vi "Arbitrary Shape Lowpass Filter Design.vi"() -> ()   [LabVIEW 2023]
doc: "Demonstrates how to design an arbitraty shape lowpass filter with two different methods. This example uses the DFD Remez Design VI to design a finite impulse response (FIR) arbitrary shape filter. This example also uses the DFD Least Pth Norm Design VI to design an infinite impulse response (IIR) arbitraty shape filter. You can see that the two filter designs are approximating the same ideal magnitude response.\n\nComplete the following steps to use this VI.\n1) Verify that this VI shows the <B>Remez Method</B> page.\n2) Run the VI and observe the magnitude response.\n3) Switch to the <B>Least Pth Norm Method</B> page.\n4) Run the VI again and observe the new magnitude response. Notice that the new magnitude response is similar to the previous one.\n5) Compare the specification settings on the <B>Remez Method</B> and <B>Least Pth Norm Method</B> pages and learn how to specify the same ideal magnitude response for different filter design methods."
uses:
  <vilib>/addons/Digital Filter Design/_LpNorm.llb/dfd_Lp Norm Filter Type.ctl
  <vilib>/addons/Digital Filter Design/_Objects.llb/DFD Adv Band Spec.ctl
  <vilib>/addons/Digital Filter Design/_REMEZ.llb/remez_fir filter type.ctl
  <vilib>/addons/Digital Filter Design/Design.llb/DFD Least Pth Norm Design by Newton.vi
  <vilib>/addons/Digital Filter Design/Analysis.llb/DFD Plot Freq Response (Linear-Spaced).vi
  <vilib>/addons/Digital Filter Design/NI_DigFilterLicensed.lvlib
panel:
  out "Error Message":string
  in  "Tab Control":enum32{"Remez Method", "Least Pth Norm Method"}(tab)
  in  "Sampling Frequency [Hz]":dbl=1.0 format="%.2f"
  in  "Filter Type":T1=enum."Minimum Phase"
  in  "Order":i32=40
  in  "Band Specifications":T2[](array[typedef])=[{"band specification"=[{"freq"=0.0, "amplitude"=1.0, "weight"=1.0}, {"freq"=0.1, "amplitude"=2.0, "weight"=1.0}, {"freq"=0.25, "amplitude"=1.0, "weight"=1.0}], "ripple constraint"=0.0}, {"band specification"=[{"freq"=0.3, "amplitude"=0.0, "weight"=1.0}, {"freq"=0.5, "amplitude"=0.0, "weight"=1.0}], "ripple constraint"=0.0}]
  in  "Band Specifications":T3(array[cluster])=[{"frequency point"=[{"frequency"=0.0, "magnitude"=1.0, "weight"=1.0, "phase"=0.0}, {"frequency"=0.1, "magnitude"=2.0, "weight"=1.0, "phase"=0.0}, {"frequency"=0.25, "magnitude"=1.0, "weight"=1.0, "phase"=0.0}]}, {"frequency point"=[{"frequency"=0.3, "magnitude"=0.0, "weight"=1.0, "phase"=0.0}, {"frequency"=0.5, "magnitude"=0.0, "weight"=1.0, "phase"=0.0}]}] {"frequency point"."weight" format="%.2f"}
  in  "Order":cluster{"numerator":i32, "denominator":i32}={"numerator"=8, "denominator"=8}
  in  "Filter Type":T4=enum."Minimum Phase"
  in  "Sampling Frequency [Hz]":dbl=1.0 format="%.2f"
  out "Magnitude Response":cluster{"f0":dbl, "df":dbl, "values":dbl[]}[](graph)
  # "Select Help>>Show Context Help and move the cursor over the VI icon for more information."
  # "freq"
  # "amplitude"
  # "weight"
  # "freq"
  # "magnitude"
  # "weight"
  # "phase"
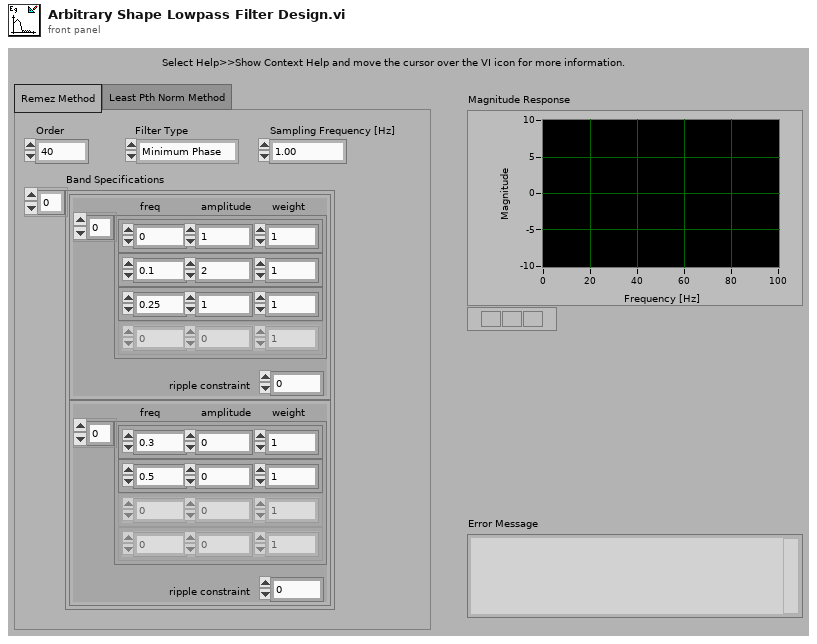
[diagram p1: front panel]
types:
  T1 = typedef "NI_DigFilterLicensed.lvlib/remez_fir filter type.ctl" = enum32{"Symmetric", "Antisymmetric", "Differentiator", "Hilbert", "Minimum Phase", "Maximum Phase"}
  T2 = typedef "NI_DigFilterLicensed.lvlib/DFD Adv Band Spec.ctl" = cluster{"band specification":cluster{"freq":dbl, "amplitude":dbl, "weight":dbl}[], "ripple constraint":dbl}
  T3 = cluster{"frequency point":cluster{"frequency":dbl, "magnitude":dbl, "weight":dbl, "phase":dbl}[]}[]
  T4 = typedef "NI_DigFilterLicensed.lvlib/dfd_Lp Norm Filter Type.ctl" = enum16{"Symmetric", "Antisymmetric", "Differentiator", "Hilbert", "Minimum Phase", "Maximum Phase"}
  T5 = typedef "NI_DigFilterLicensed.lvlib/DFD Filter Obj.ctl" = cluster{"mSRate_Fs":dbl, "mSRate_Version":string, "mSRate_Comments":string, "mSRate_OrgCoef":T6, "mSRate_CurCoef":T6, "mSRate_Quantized?":bool, "mSRate_QCoef":T6, "mSRate_QSettings":T8[], "mSRate_Order":i32, "mSRate_Scaling":cluster{"mSRate_ScaleByPowerOf2?":bool, "mSRate_ScaleType":T10}}
  T6 = typedef "NI_DigFilterLicensed.lvlib/DFD Filter Coef.ctl" = cluster{"type":T7, "gain":dbl, "coef a (k)":dbl[], "coef b (v)":dbl[]}
  T7 = typedef "NI_DigFilterLicensed.lvlib/DFD Filter Structure Type Selector.ctl" = enum16{"Undefined", "FIR Direct Form", "FIR Direct Form Transposed", "FIR Symmetric", "FIR Antisymmetric", "IIR Direct Form I", "IIR Direct Form I Transposed", "IIR Direct Form II", "IIR Direct Form II Transposed", "IIR Cascaded Second Order Sections Form I", "IIR Cascaded Second Order Sections Form I Transposed", "IIR Cascaded Second Order Sections Form II", "IIR Cascaded Second Order Sections Form II Transposed", "Lattice Allpass (basic sections)", "Lattice Allpass (one multiplier sections)", "Lattice Allpass (normalized sections)", "Lattice AR (basic sections)", "Lattice AR (one multiplier sections)", "Lattice AR (normalized sections)", "Lattice MA (minimum phase)", "Lattice MA (maximum phase)", "Lattice ARMA (basic sections)", "Lattice ARMA (one multiplier sections)", "Lattice ARMA (normalized sections)"}
  T8 = typedef "NI_DigFilterLicensed.lvlib/dfd_Internal Quantization Settings.ctl" = cluster{"source":T9, "wl":i16, "iwl":i16, "overflow mode":enum16{"Saturation", "Wrap"}, "rounding mode":enum16{"Nearest", "Truncation"}, "signed?":bool}
  T9 = typedef "NI_DigFilterLicensed.lvlib/dfd_Internal Quantization Srcs.ctl" = u16
  T10 = typedef "NI_DigFilterLicensed.lvlib/DFD Coef Norm Type.ctl" = enum16{"No Norm", "Time Domain 1-Norm", "Time Domain 2-Norm", "Time Domain Inf-Norm"}
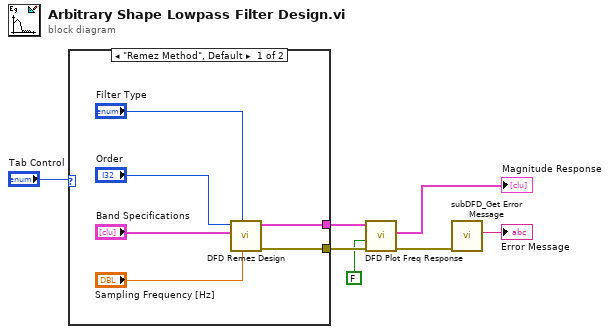
[diagram p0: block diagram]
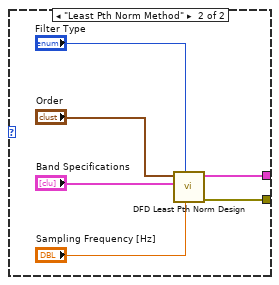
[diagram p2: hidden frame]
diagram:
  n1 = case shown="\"Remez Method\", Default" "Tab Control" {
    tunnel: [w13 w18] -> w6
    tunnel: [w12 w17] -> w5
    frame "Remez Method", Default {
      n2 = call <vilib>:"DFD Remez Design.vi"("fs [Hz]"="Sampling Frequency [Hz]", "filter type"="Filter Type", "band specs"="Band Specifications", "order"="Order") -> ("error out"=w12:errorcluster, "filter out"=w13:T5)  [unwired: 3 in, 3 out]
    }
    frame "Least Pth Norm Method" {
      n3 = call-poly <vilib>:"DFD Least Pth Norm Design.vi"("fs [Hz]"="Sampling Frequency [Hz]", "filter type"="Filter Type", "band specs"="Band Specifications", "order"="Order") -> ("error out"=w17:errorcluster, "filter out"=w18:T5)  [unwired: 4 in, 2 out]
    }
  }
  n4 = call-poly <vilib>:"DFD Plot Freq Response.vi"("error in (no error)"=w5, "dB on? (T)"=FALSE, "filter in"=w6) -> ("error out"=w1:errorcluster, "magnitude response"=→"Magnitude Response":cluster{"f0":dbl, "df":dbl, "values":dbl[]}[])  [unwired: 5 in, 2 out]
  n5 = call <vilib>:"subDFD_Get Error Message.vi"("error in (no error)"=w1) -> ("Error Message"=→"Error Message":string)  [unwired: 10 out]
